vi "AngleToWristEncoder.vi"(11 "angle(deg)":dbl) -> (3 "encoderPulses":i32)   [LabVIEW 2018]
uses:
  Arm Constants.vi
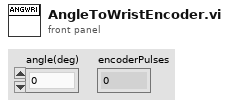
[diagram p1: front panel]
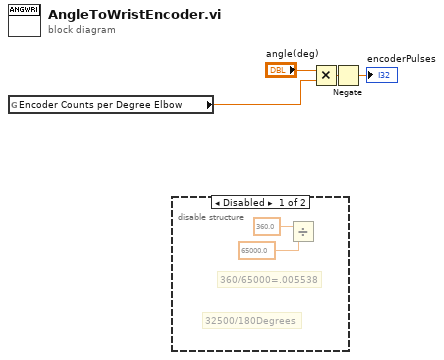
[diagram p0: block diagram]
diagram:
  n1 = global read "Arm Constants.vi" "Encoder Counts per Degree Elbow"() -> (w3:dbl)
  n2 = disable-structure shown="Disabled" {
    frame Disabled {
      # "360/65000=.005538"
      # "32500/180Degrees"
      n3 = Divide(x=360.0, y=65000.0) -> ()  [unwired: 1 out]
    }
    frame Enabled {
    }
  }
  n4 = Multiply(x="angle(deg)", y=w3) -> (x*y=w2:dbl)
  n5 = Negate(x=w2) -> (-x=→"encoderPulses":dbl)
